vi "WebView.Tabulator_Init.vi"(8 "Error In":errorcluster, 10 "WebView2 Control in":refnum<k24>(container), 11 "Object in":refnum<class "WebView.Tabulator.lvclass">) -> (0 "Error Out":errorcluster, 3 "object out":refnum<class "WebView.Tabulator.lvclass">)   [LabVIEW 2020, in "WebView.Tabulator.lvclass"]
uses:
  WebView.Tabulator.lvclass
  WebView.Tabulator.lvclass/WebView.Tabulator.ctl
  E:/Git/WebView-Components/Source/Component_class/Component.lvclass
  E:/Git/WebView-Components/Source/WebView.Tabulator_class/WebView.Tabulator.lvclass
  Component_class/Component.lvclass
  <vilib>/sklein/WebView2/Webview2 Lib/WebView2 Control Object/WebView2 Control.lvclass
  <vilib>/sklein/WebView2/Libs/Microsoft.Web.WebView2.WinForms.dll
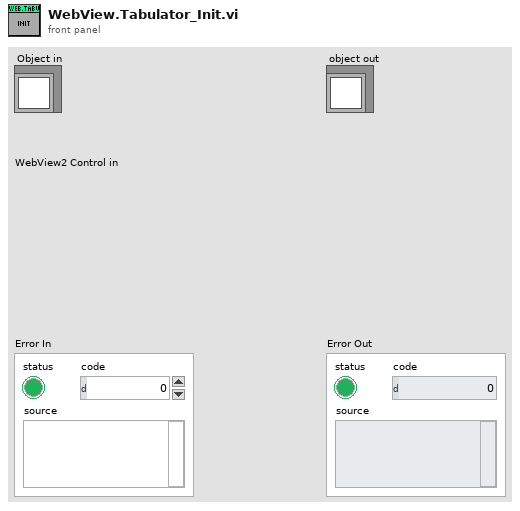
[diagram p1: front panel]
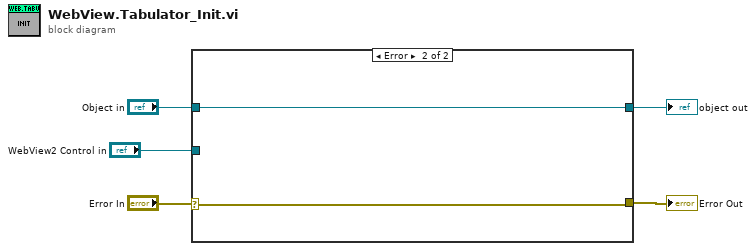
[diagram p0: block diagram]
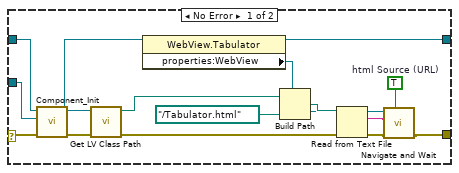
[diagram p2: hidden frame]
diagram:
  n1 = case shown="Error" "Error In" {
    selector: "Error In" -> [w20 w22]
    tunnel: [w6 w22] -> w4
    tunnel: "WebView2 Control in" -> [w14 _]
    tunnel: [w12 w21] -> w2
    tunnel: "Object in" -> [w11 w21]
    frame No Error {
      w7 = TRUE  # html Source (URL)
      n2 = call "Component_Init.vi"("Error In"=w20, "WebView2"=w14, "object in"=w11) -> ("Error Out"=w15:errorcluster, "object out"=w13:refnum<class "WebView.Tabulator.lvclass">)  [unwired: 7 in]
      n3 = call <vilib>:"Get LV Class Path.vi"("error in (no error)"=w15, "object"=w13) -> ("error out"=w16:errorcluster, "class path"=w19:path)  [unwired: 8 in]
      n4 = property class="WebView.Tabulator"(reference=w13) -> (reference out=w12:refnum<class "WebView.Tabulator.lvclass">, "properties:WebView"=w10:refnum<class "WebView2 Control.lvclass">)  [unwired: 1 in, 1 out]
      n5 = Build Path(base path=w19, name or relative path=path "../Tabulator.html") -> (appended path=w17:path)
      n6 = Read from Text File(file (use dialog)=w17, error in=w16) -> (text=w8:string, error out=w9:errorcluster)  [unwired: 2 in, 2 out]
      n7 = call <vilib>:"Navigate and Wait.vi"("html Source (URL)"=w7, "error in (no error)"=w9, "Source"=w8, "WebView2 Control in"=w10) -> ("error out"=w6:errorcluster)  [unwired: 5 in, 2 out]
    }
    frame Error {
    }
  }
  "object out" <- w2
  "Error Out" <- w4
